vi "UE FGV.vi"(7 "UE Ctls":T2, 8 "error in (no error)":errorcluster, 11 "event data":T1) -> (0 "error out":errorcluster, 3 "UE Dataset":refnum<user-event>)   [LabVIEW 2021, in "User Event.lvlib"]
uses:
  User Event.lvlib
  UE Control.ctl
  UE Dataset.ctl
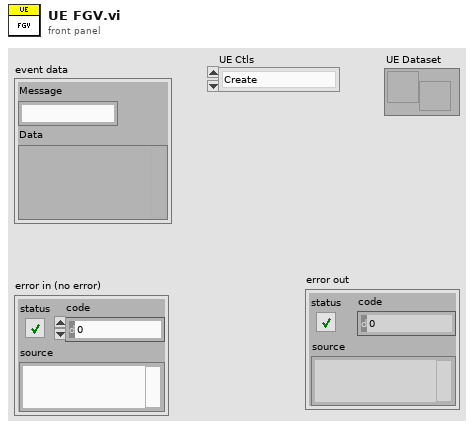
[diagram p1: front panel]
types:
  T1 = typedef "User Event.lvlib/UE Dataset.ctl" = cluster{"Message":string, "Data":variant}
  T2 = typedef "User Event.lvlib/UE Control.ctl" = enum16{"Create", "Get", "Generate", "Destroy"}
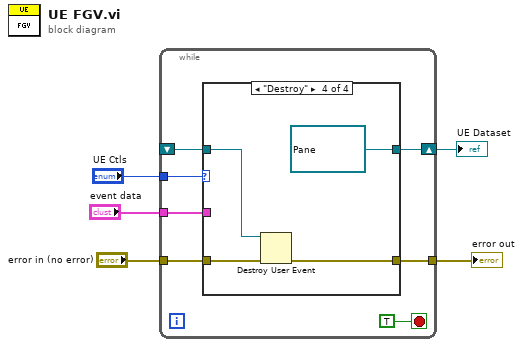
[diagram p0: block diagram]
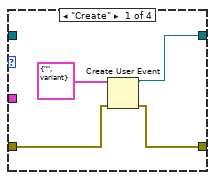
[diagram p2: hidden frame]
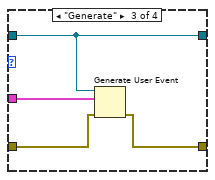
[diagram p4: hidden frame]
diagram:
  n1 = while {
    tunnel: "error in (no error)" -> [w11]
    tunnel: "UE Ctls" -> [w10]
    tunnel: [w9] -> w3
    shift-right: [w8] -> w2
    shift-left: _ -> [w7]
    tunnel: "event data" -> [w6]
    stop <- TRUE stop-if-true
    n2 = case shown="\"Destroy\"" w10 {
      tunnel: w11 -> [w15 w17 w22 w25]
      tunnel: [w14 w17 w21 w24] -> w9
      tunnel: [w13 w18 w19 refnum<user-event> refnum ("UE Dataset")] -> w8
      tunnel: w7 -> [_ w18 w19 w26]
      tunnel: w6 -> [_ _ w20 _]
      frame "Create" {
        n3 = Create User Event(user event datatype=T1 {"Message"="", "Data"=variant} ("UE Dataset"), error in=w15) -> (user event=w13:refnum<user-event>, error out=w14:errorcluster)
      }
      frame "Get", Default {
      }
      frame "Generate" {
        n4 = Generate User Event(user event=w19, event data cluster=w20, error in=w22) -> (error out=w21:errorcluster)  [unwired: 1 in, 1 out]
      }
      frame "Destroy" {
        n5 = Destroy User Event(user event=w26, error in=w25) -> (error out=w24:errorcluster)
      }
    }
  }
  "error out" <- w3
  "UE Dataset" <- w2
